vi "SOS main.vi"() -> ()   [LabVIEW 2017]
uses:
  <extravilib>/ChannelInstances/Lossy Stream-t'SSL Referee Game Status.ctl'.lvlib
  <extravilib>/ChannelInstances/Lossy Stream-t'AI Input.ctl'.lvlib
  SSL Referee Game Status.ctl
  SSL Detection Robot.ctl
  SSL Detection Ball.ctl
  SSL Detection Frame.ctl
  SSL/SSL Field State.ctl
  <extravilib>/ChannelInstances/Lossy Stream-t'SSL Field State.ctl'.lvlib
  <extravilib>/ChannelInstances/Lossy Stream-a[.](u8).lvlib
  <vilib>/Analysis/Matrix/Datatypes/RealMatrix.ctl
  <vilib>/Analysis/Matrix/NI_Matrix.lvlib
  <extravilib>/ChannelInstances/Lossy Stream-c(a[.](c(c(dbl,dbl,dbl,dbl,dbl),c(dbl,dbl,dbl,dbl,dbl),c(dbl,dbl,dbl,dbl,dbl,u32),u32,u32)),t'Events.ctl').lvlib
  <extravilib>/ChannelInstances/Lossy Stream-c(t'AI Ball.ctl',a[.](c(c(dbl,dbl,dbl,dbl,dbl),c(dbl,dbl,dbl,dbl,dbl),c(dbl,dbl,dbl,dbl,dbl,u32),u32,u32))).lvlib
  <extravilib>/ChannelInstances/Lossy Stream-a[.](i32).lvlib
  Filters/Estimadores.ctl
  Control/SSL UDP Address.ctl
  Control/File Player.ctl
  Control/SSL Data Control.ctl
  Intel/Command Enum.ctl
  DrawTargets.ctl
  grSim/grSim RobotReplacement.ctl
  grSim/grSim_BallReplacement.ctl
  Core/AI Ball.ctl
panel:
  in  "Tab Control 2":T1(tab)
  out "2D Picture":picture
  out "Kick Error Histogram":cluster{dbl[], dbl[]}(graph)
  out "Goalie Error Histogram":cluster{dbl[], dbl[]}(graph)
  out "Heatmap by ID":picture
  in  "ID":i32
  in  "Kalman Error\nID":i32
  out "Kalman Error Histogram":cluster{dbl[], dbl[]}(graph)
  in  "element":T3
  in  "grid y":dbl=30.0 format="%#_13g"
  in  "grid x":dbl=45.0 format="%#_13g"
  in  "Draw Targets?":T4={"Attacker"=TRUE, "Striker"=TRUE, "Goalie"=TRUE, "Defender"=TRUE, "kick"=TRUE, "Est Ball"=TRUE, "Est Robot"=FALSE}
  in  "SSL Data":T5={"Modo"=TRUE, "SSL UDP RX"={"Port:"=10020, "Server IP:"="224.5.23.2", "Local IP:"="", "RX"=TRUE}, "RefBox UDP RX"={"Port:"=10003, "Server IP:"="224.5.23.1", "Local IP:"="", "RX"=TRUE}, "Reprodução de Arquivo"={"file path (use dialog)"=path "E:/Media/2016-07-01_cmdragons_immortals.log", "size (in bytes)"=0, "offset (in bytes)"=0, "Slide"=0.0, "Play"=FALSE, "Time Stamp"=timestamp(0 s since 1904-01-01), "Playing"=FALSE}, "SSL UDP SOS RX IA_State"={"Port:"=10030, "Server IP:"="224.5.23.2", "Local IP:"="", "RX"=TRUE}, "SSL UDP SOS RX  Enemy State"={"Port:"=10020, "Server IP:"="224.5.23.2", "Local IP:"="224.5.23.2", "RX"=FALSE}} {"Reprodução de Arquivo"."Time Stamp" format="%<%.3X %x>T"; "Reprodução de Arquivo"."Slide" min=0 max=1 scale=0.0..1.0; "Reprodução de Arquivo"."offset (in bytes)" format="%.3p"; "Reprodução de Arquivo"."size (in bytes)" format="%.3p"}
  out "error out 5":errorcluster
  out "error out 3":errorcluster
  out "IA command":T8
  in  "ignora esquerda?":bool
  in  "ignora lado?":bool
  in  "Defense stretch":i32=300
  in  "Defense radius":i32=460
  in  "Estimador":T9=enum."Kalman"
  out "Total Delay":dbl format="%#.5g"
  in  "Goalie":string(combo)="0"
  in  "Command":string(combo)="Auto"
  in  "Time":enum16{"Azul", "Amarelo"}(ring) caption="Enum"
  in  "Lado":enum16{"Esquerdo", "Direito"}(ring) caption="Enum"
  in  "Tab Control":enum32{"RX Info", "TX info", "AI Parameters"}(tab)
  out "Game Status":T10={"Stage"="Normal First Half Pre", "Command"="Stop", "Time Left"=0.0, "Yellow Team"="", "Blue Team"="", "Yellow Score"=0, "Blue Score"=0, "Yellow Red Cards"=0, "Blue Red Cards"=0, "Yellow Yellow Cards"=0, "Blue Yellow Cards"=0, "Yellow Timeouts Left"=0, "Blue Timeouts Left"=0, "Yellow Timeout Remaining"=0.0, "Blue Timeout Remaining"=0.0, "Yellow Goalie Id"=0, "Blue Goalie Id"=0, "Time"=timestamp(2082758400 s since 1904-01-01)} {"Time" format="%<%.3X %x>T"; "Blue Timeout Remaining" format="%<%M:%S>t"; "Yellow Timeout Remaining" format="%<%M:%S>t"; "Time Left" format="%<%M:%S>t"}
  in  "Serial TX":bool
  in  "UDP TX":bool=TRUE
  in  "Address:":string="127.0.0.1"
  in  "Port:":u16=20011
  in  "Porta:":refnum<visa-resource-name>
  out "Comm FPS":dbl
  in  "replace active":bool
  in  "grSim replacement":cluster{"robots":T11[], "ball":T12}={"robots"=[{"x"=0.0, "y"=-450.0, "dir"=0.0, "yellowteam"=FALSE, "id"=0}, {"x"=0.0, "y"=-270.0, "dir"=0.0, "yellowteam"=FALSE, "id"=1}, {"x"=0.0, "y"=-90.0, "dir"=0.0, "yellowteam"=FALSE, "id"=2}, {"x"=0.0, "y"=90.0, "dir"=0.0, "yellowteam"=FALSE, "id"=3}, {"x"=0.0, "y"=270.0, "dir"=0.0, "yellowteam"=FALSE, "id"=4}, {"x"=0.0, "y"=450.0, "dir"=0.0, "yellowteam"=FALSE, "id"=5}], "ball"={"x"=0.0, "y"=0.0, "vx"=0.0, "vy"=0.0}}
  # "UDP"
  # "LOG"
  # "Score"
  # "Red Cards"
  # "Yellow Cards"
  # "Timeouts Left"
  # "Timeout Remaining"
  # "Goalie ID"
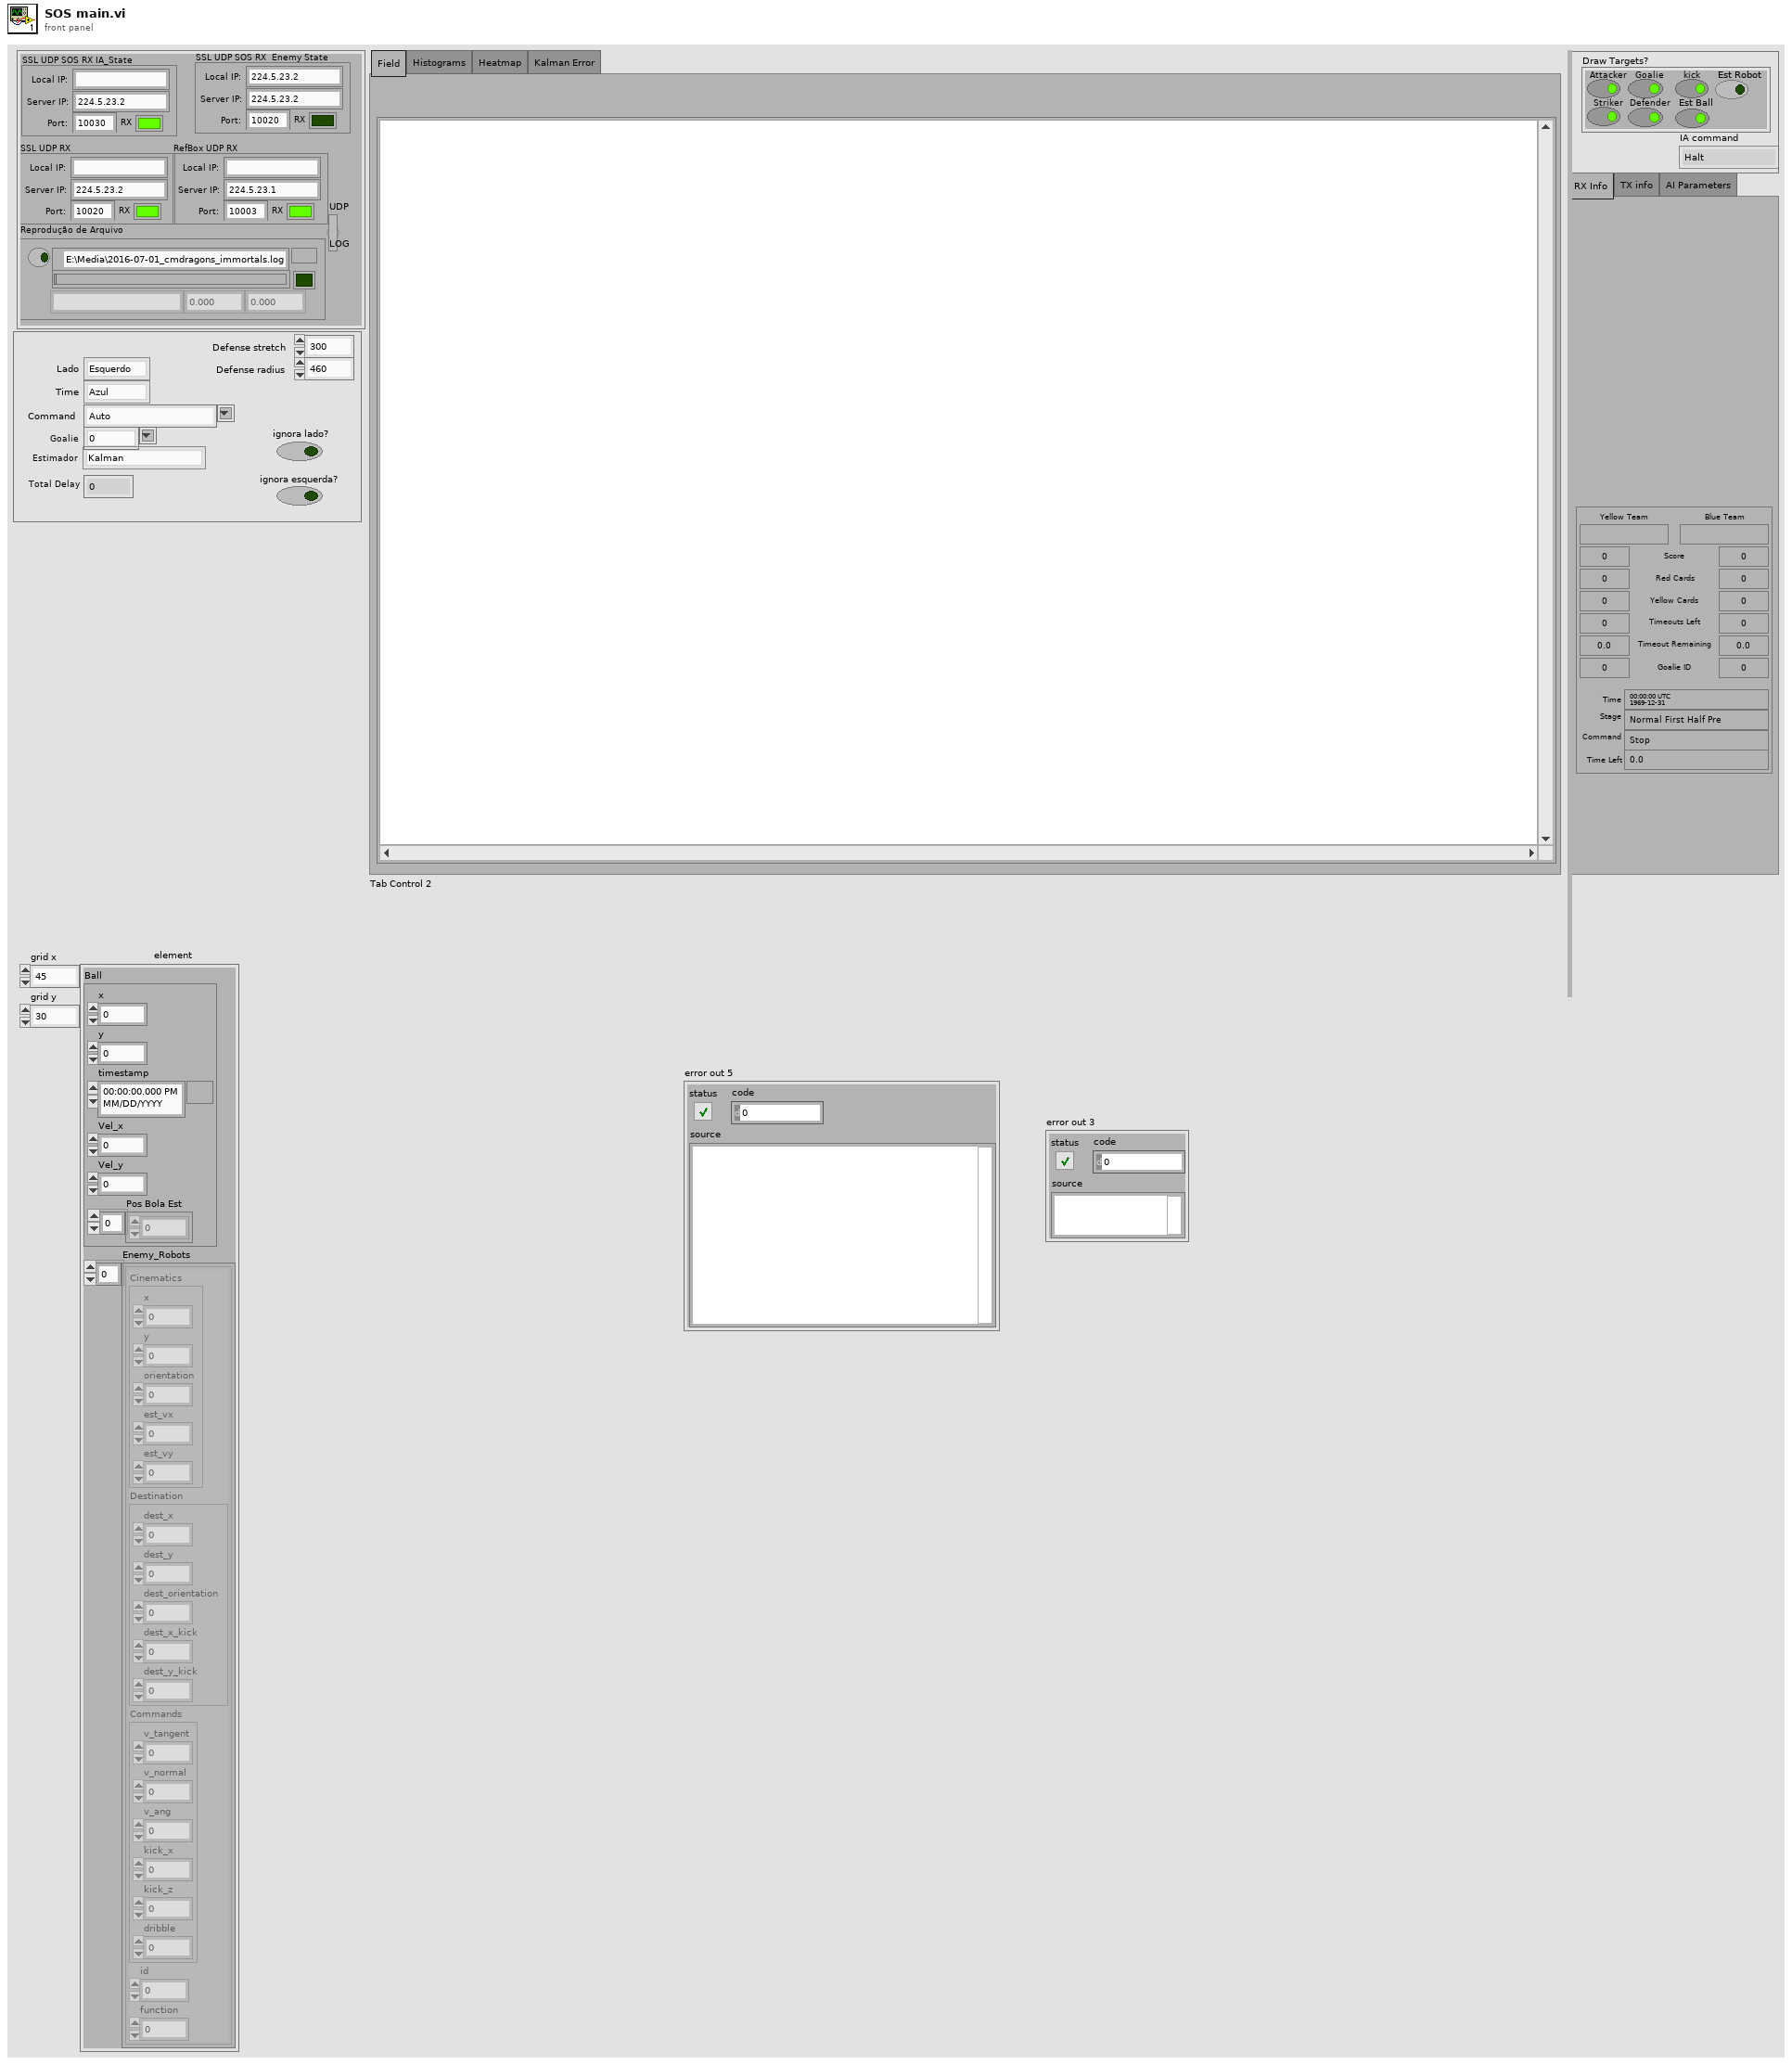
[diagram p1: front panel]
types:
  T1 = enum32{"Field", "Histograms", "Heatmap", "Kalman Error"}
  T2 = typedef "AI Ball.ctl" = cluster{"x":dbl, "y":dbl, "timestamp":timestamp, "Vel_x":dbl, "Vel_y":dbl, "Pos Bola Est":dbl[]}
  T3 = cluster{"Ball":T2, "Enemy_Robots":cluster{"Cinematics":cluster{"x":dbl, "y":dbl, "orientation":dbl, "est_vx":dbl, "est_vy":dbl}, "Destination":cluster{"dest_x":dbl, "dest_y":dbl, "dest_orientation":dbl, "dest_x_kick":dbl, "dest_y_kick":dbl}, "Commands":cluster{"v_tangent":dbl, "v_normal":dbl, "v_ang":dbl, "kick_x":dbl, "kick_z":dbl, "dribble":u32}, "id":u32, "function":u32}[]}
  T4 = typedef "DrawTargets.ctl" = cluster{"Attacker":bool, "Striker":bool, "Goalie":bool, "Defender":bool, "kick":bool, "Est Ball":bool, "Est Robot":bool}
  T5 = typedef "SSL Data Control.ctl" = cluster{"Modo":bool, "SSL UDP RX":T6, "RefBox UDP RX":T6, "Reprodução de Arquivo":T7, "SSL UDP SOS RX IA_State":T6, "SSL UDP SOS RX  Enemy State":T6}
  T6 = typedef "SSL UDP Address.ctl" = cluster{"Port:":u16, "Server IP:":string, "Local IP:":string, "RX":bool}
  T7 = typedef "File Player.ctl" = cluster{"file path (use dialog)":path, "size (in bytes)":i64, "offset (in bytes)":i64, "Slide":sgl, "Play":bool, "Time Stamp":timestamp, "Playing":bool}
  T8 = typedef "Command Enum.ctl" = enum16{"Halt", "Stop", "Force Start", "PKA Normal Start", "Prepare Kickoff Ally", "PKE Normal Start", "Prepare Kickoff Enemy", "Prepare Penalty Ally", "PPA Normal Start", "Prepare Penalty Enemy", "PPE Normal Start", "Direct Free Enemy", "Direct Free Ally", "Indirect Free Enemy", "Indirect Free Ally", "Timeout Enemy", "Timeout Ally", "Goal Enemy", "Goal Ally", "Ball Placement Enemy", "Ball Placement Ally", "Normal Half Time", "Extra Time Break", "Extra Half Time", "None", "Post Game"}
  T9 = typedef "Estimadores.ctl" = enum16{"Nenhum", "Simples", "Kalman"}
  T10 = typedef "SSL Referee Game Status.ctl" = cluster{"Stage":string, "Command":string, "Time Left":dbl, "Yellow Team":string, "Blue Team":string, "Yellow Score":u32, "Blue Score":u32, "Yellow Red Cards":u32, "Blue Red Cards":u32, "Yellow Yellow Cards":u32, "Blue Yellow Cards":u32, "Yellow Timeouts Left":u32, "Blue Timeouts Left":u32, "Yellow Timeout Remaining":dbl, "Blue Timeout Remaining":dbl, "Yellow Goalie Id":u32, "Blue Goalie Id":u32, "Time":timestamp}
  T11 = typedef "grSim RobotReplacement.ctl" = cluster{"x":dbl, "y":dbl, "dir":dbl, "yellowteam":bool, "id":u32}
  T12 = typedef "grSim_BallReplacement.ctl" = cluster{"x":dbl, "y":dbl, "vx":dbl, "vy":dbl}
  T13 = typedef "Lossy Stream-a[.](u8).lvlib/)Channel.ctl" = refnum<queue>
  T14 = typedef "Lossy Stream-c(t'AI Ball.ctl',a[.](c(c(dbl,dbl,dbl,dbl,dbl),c(dbl,dbl,dbl,dbl,dbl),c(dbl,dbl,dbl,dbl,dbl,u32),u32,u32))).lvlib/)Channel.ctl" = refnum<queue>
  T15 = typedef "SSL Field State.ctl" = cluster{"Detection Frame Out":T16, "Field Size Out":cluster{"line_width":u32, "field_length":u32, "field_width":u32, "boundary_width":u32, "referee_width":u32, "goal_width":u32, "goal_depth":u32, "goal_wall_width":u32, "center_circle_radius":u32, "defense_radius":u32, "defense_stretch":u32, "free_kick_from_defense_dist":u32, "penalty_spot_from_field_line_dist":u32, "penalty_line_from_spot_dist":u32}, "Received Time Stamp":timestamp}
  T16 = typedef "SSL Detection Frame.ctl" = cluster{"frame_number":u32, "t_capture":dbl, "t_sent":dbl, "camera_id":u32, "robots_yellow":T17[], "robots_blue":T17[], "balls":T19[], "Valid":bool, "Time Stamp":timestamp}
  T17 = typedef "SSL Detection Robot.ctl" = cluster{"x":sgl, "robot_id":u32, "confidence":sgl, "y":sgl, "orientation":sgl, "pixel_x":sgl, "pixel_y":sgl, "height":sgl, "Valid":bool, "Time Stamp":timestamp, "x_k|k":T18, "Pk|k":T18, "Previous Time Stamp":timestamp, "R":T18}
  T18 = typedef "NI_Matrix.lvlib/RealMatrix.ctl" = dbl[][]
  T19 = typedef "SSL Detection Ball.ctl" = cluster{"x":sgl, "area":u32, "confidence":sgl, "y":sgl, "z":sgl, "pixel_x":sgl, "pixel_y":sgl, "Valid":bool, "Time Stamp":timestamp, "x_k|k":T18, "Pk|k":T18, "Id":u32, "Previous Time Stamp":timestamp, "R":T18}
  T20 = cluster{"line_width":u32, "field_length":u32, "field_width":u32, "boundary_width":u32, "referee_width":u32, "goal_width":u32, "goal_depth":u32, "goal_wall_width":u32, "center_circle_radius":u32, "defense_radius":u32, "defense_stretch":u32, "free_kick_from_defense_dist":u32, "penalty_spot_from_field_line_dist":u32, "penalty_line_from_spot_dist":u32}
  T21 = typedef "Lossy Stream-t'SSL Field State.ctl'.lvlib/)Channel.ctl" = refnum<queue>
  T22 = typedef "Events.ctl" = cluster{"Touch":bool, "Ball out":bool, "id touch":dbl, "Ball out of \nVision":bool, "Ball inside \nGoalie area":bool, "Robot not responding":bool, "Robots responding status":dbl[], "Enemy Ball \nPossession":bool, "Pass State":bool, "id end of pass":dbl, "Kick":bool, "Id ini Possession":dbl, "Ball Possesion":bool, "Id Possesion":dbl}
  T23 = cluster{"Our_Robots":cluster{"Cinematics":cluster{"x":dbl, "y":dbl, "orientation":dbl, "est_vx":dbl, "est_vy":dbl}, "Destination":cluster{"dest_x":dbl, "dest_y":dbl, "dest_orientation":dbl, "dest_x_kick":dbl, "dest_y_kick":dbl}, "Commands":cluster{"v_tangent":dbl, "v_normal":dbl, "v_ang":dbl, "kick_x":dbl, "kick_z":dbl, "dribble":u32}, "id":u32, "function":u32}[], "Events":T22}
  T24 = typedef "Lossy Stream-c(a[.](c(c(dbl,dbl,dbl,dbl,dbl),c(dbl,dbl,dbl,dbl,dbl),c(dbl,dbl,dbl,dbl,dbl,u32),u32,u32)),t'Events.ctl').lvlib/)Channel.ctl" = refnum<queue>
  T25 = typedef "SSL Referee.ctl" = cluster{"packet_\ntimestamp":u64, "stage":u64, "stage_time_left":i32, "command ":u64, "command_\ncounter ":u32, "command_\ntimestamp":u64, "yellow team info":T26, "blue team info":T26, "Point":cluster{"x":sgl, "y":sgl}}
  T26 = typedef "SSL Referee Team Info.ctl" = cluster{"name":string, "score":u32, "red_cards":u32, "yellow_cards_time":u32[], "yellow_cards":u32, "timeout":u32, "timeout_times":u32, "goalie":u32}
  T27 = typedef "Lossy Stream-t'SSL Referee Game Status.ctl'.lvlib/)Channel.ctl" = refnum<queue>
  T28 = typedef "AI Input.ctl" = cluster{"our_robots":T29[], "enemy_robots":T29[], "balls":T2[], "geometry":T32, "IA Judge":T33, "Received Timestamp":timestamp, "Events":T22}
  T29 = typedef "AI Robot.ctl" = cluster{"id":u32, "function":T30, "x":dbl, "y":dbl, "orientation":dbl, "v_tangent":dbl, "v_normal":dbl, "v_ang":dbl, "kick_x":dbl, "kick_z":dbl, "dribble":bool, "Timestamp":timestamp, "dest_x":dbl, "dest_y":dbl, "dest_orientation":dbl, "estimatives":cluster{"est_v_tangent":dbl, "est_v_normal":dbl, "est_vx":dbl, "est_vy":dbl, "Pos Robot Est":dbl[]}, "dest_x_kick":dbl, "dest_y_kick":dbl, "Gap Coord":dbl[], "States":T31}
  T30 = typedef "Functions Enum.ctl" = enum16{"Attacker", "Goalie", "Defender", "Striker", "Goto 0", "Dummy", "Kicker", "ZigZag"}
  T31 = typedef "AttackerStates.ctl" = enum16{"Pass", "GoToTangent", "BallGetting", "GoToKick", ""}
  T32 = typedef "Field Size.ctl" = cluster{"line_width":u32, "field_length":u32, "field_width":u32, "boundary_width":u32, "referee_width":u32, "goal_width":u32, "goal_depth":u32, "goal_wall_width":u32, "center_circle_radius":u32, "defense_radius":u32, "defense_stretch":u32, "free_kick_from_defense_dist":u32, "penalty_spot_from_field_line_dist":u32, "penalty_line_from_spot_dist":u32}
  T33 = typedef "AI Judge.ctl" = cluster{"stage":string, "command":string, "our_goalie_id":dbl, "enemy_goalie_id":dbl, "command enum":T8, "Time":enum16{"Azul", "Amarelo"}}
  T34 = typedef "Lossy Stream-a[.](i32).lvlib/)Channel.ctl" = refnum<queue>
  T35 = typedef "Lossy Stream-t'AI Input.ctl'.lvlib/)Channel.ctl" = refnum<queue>
  T36 = typedef "grSim Robot Command.ctl" = cluster{"id":u32, "kickspeedx":sgl, "kickspeedz":sgl, "veltangent":sgl, "velnormal":sgl, "velangular":sgl, "spinner":bool, "wheelspeed":bool, "wheel1":sgl, "wheel2":sgl, "wheel3":sgl, "wheel4":sgl}
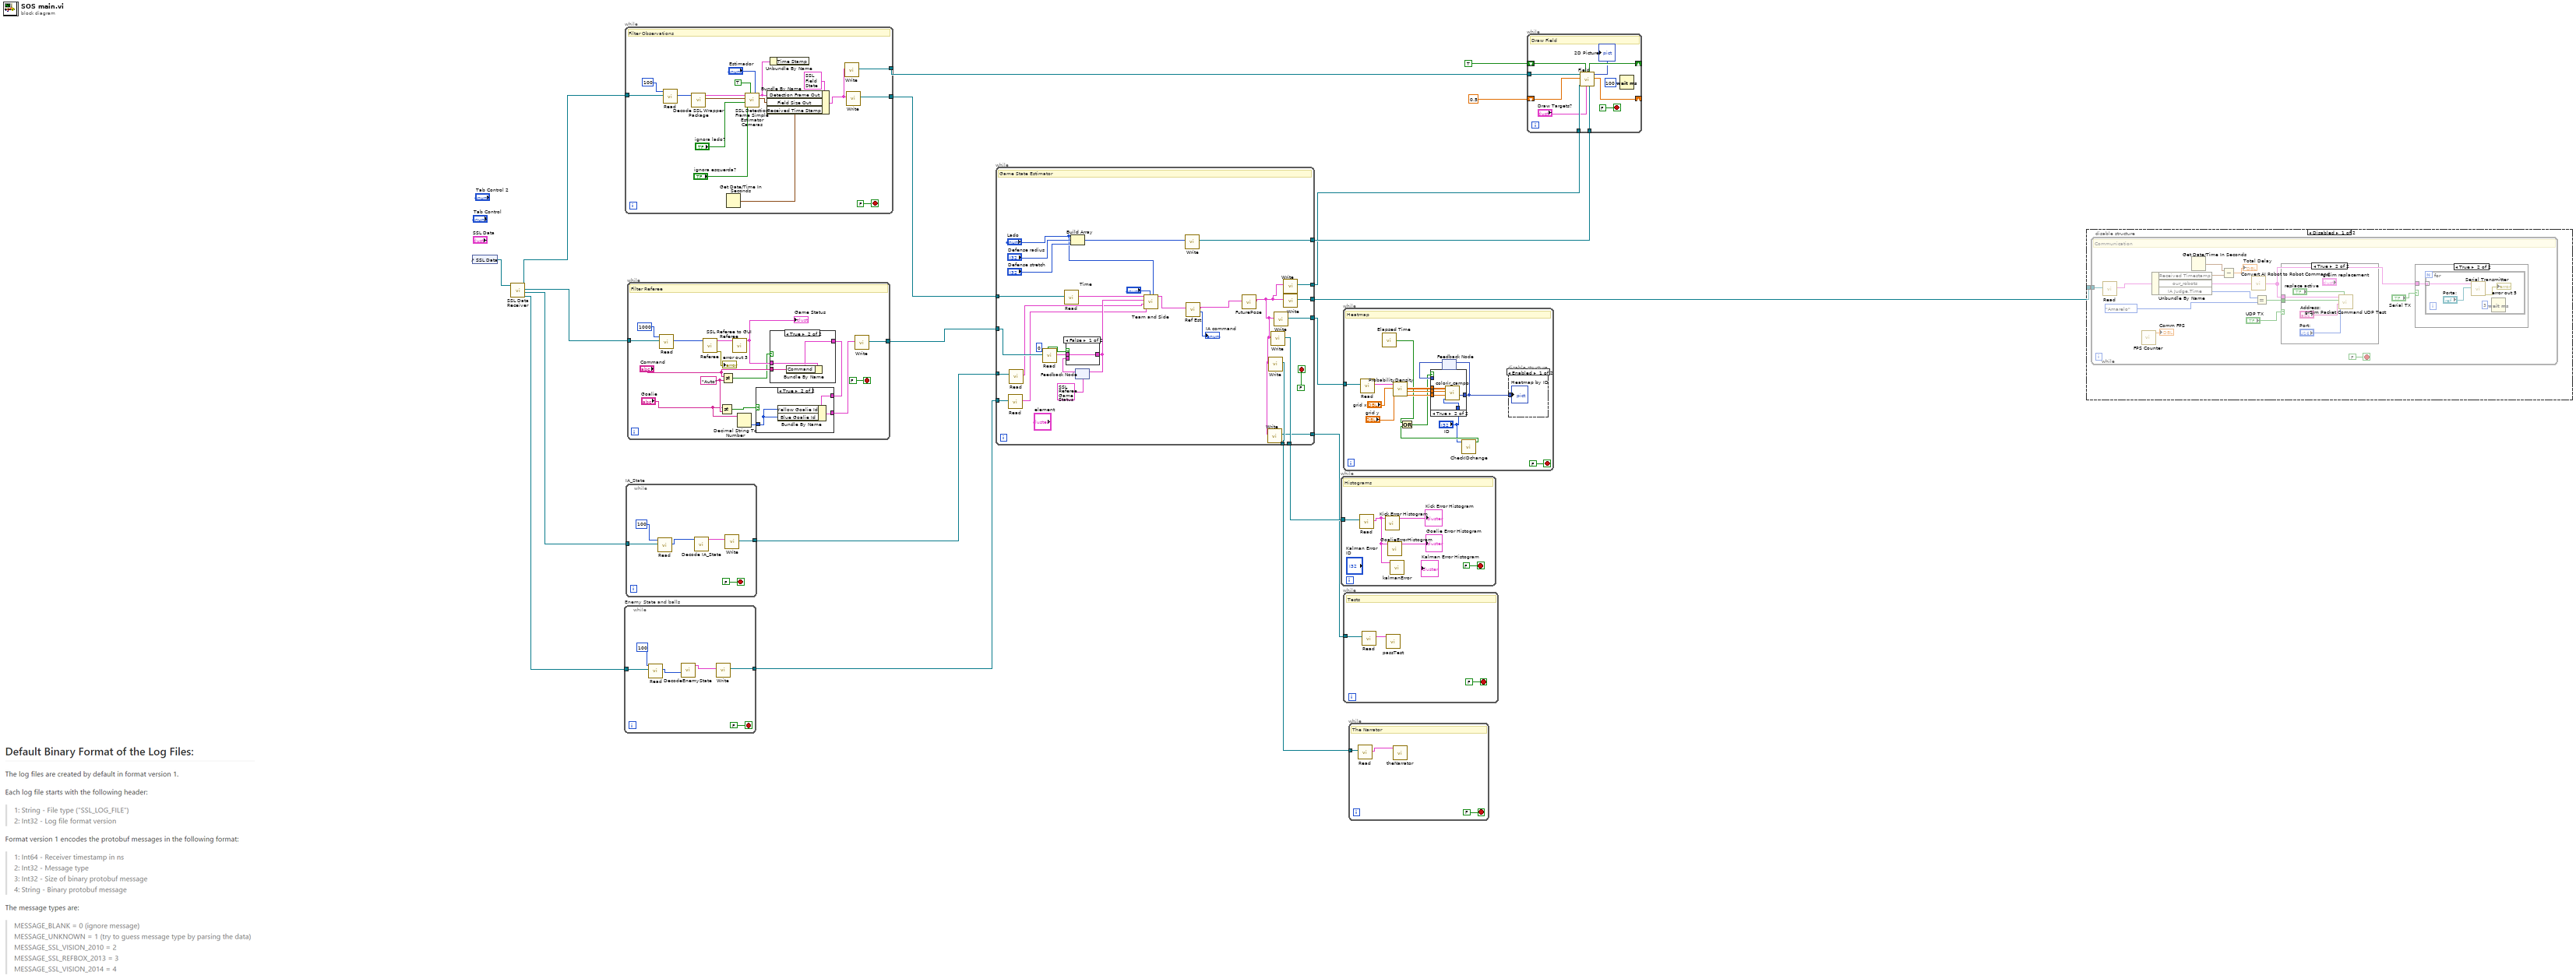
[diagram p0: block diagram]
diagram:
  n1 = control-ref of="SSL Data"() -> (w9:refnum<vi>)
  n2 = call "SSL Data Receiver.vi"("SSL Data"=w9) -> ("Enemy_State"=w10:T13, "IA_State"=w11:T13, "SSL RefBox"=w14:T13, "SSL Vision"=w15:T13)  [unwired: 7 in]
  n3 = while "Enemy State and balls" {
    tunnel: w10 -> [w23]
    tunnel: [w20] -> w7
    stop <- FALSE stop-if-true
    n4 = call <extravilib>:"Read.vi"("channel"=w23, "timeout in ms (-1)"=100) -> ("element"=w24:u8[])  [unwired: 4 in, 5 out]
    n5 = call "DecodeEnemyState.vi"("array"=w24) -> ("output cluster"=w21:T3)  [unwired: 8 in, 2 out]
    n6 = call <extravilib>:"Write.vi"("element"=w21) -> ("channel"=w20:T14)  [unwired: 8 in, 2 out]
  }
  n7 = while {
    tunnel: [w27] -> w13
    tunnel: [w35] -> w17
    tunnel: w15 -> [w32]
    stop <- FALSE stop-if-true
    # "Filter Observations"
    n8 = call <extravilib>:"Read.vi"("channel"=w32, "timeout in ms (-1)"=100) -> ("element"=w31:u8[])  [unwired: 4 in, 5 out]
    n9 = call "Decode SSL Wrapper Package.vi"("unsigned byte array"=w31) -> ("Field Size"=w40:T20, "Detection Frame"=w41:T16)  [unwired: 7 in, 2 out]
    n10 = Get Date/Time In Seconds() -> (seconds since 1Jan1904=w37:timestamp)
    n11 = call "SSL Detection Frame Simple Estimator Cameras.vi"("Estimador"="Estimador", "Enable"=TRUE, "ignora esquerda?"="ignora esquerda?", "ignora lado?"="ignora lado?", "Field Size"=w40, "Detection Frame In"=w41) -> ("Field Size Out"=w36:T20, "Detection Frame Out"=w34:T16)  [unwired: 4 in]
    n12 = Bundle By Name(cluster=T15 {"Detection Frame Out"={"frame_number"=0, "t_capture"=0.0, "t_sent"=0.0, "camera_id"=0, "robots_yellow"=[], "robots_blue"=[], "balls"=[], "Valid"=FALSE, "Time Stamp"=timestamp(0 s since 1904-01-01)}, "Field Size Out"={"line_width"=0, "field_length"=0, "field_width"=0, "boundary_width"=0, "referee_width"=0, "goal_width"=0, "goal_depth"=0, "goal_wall_width"=0, "center_circle_radius"=0, "defense_radius"=0, "defense_stretch"=0, "free_kick_from_defense_dist"=0, "penalty_spot_from_field_line_dist"=0, "penalty_line_from_spot_dist"=0}, "Received Time Stamp"=timestamp(0 s since 1904-01-01)}, "Detection Frame Out"=w34, "Field Size Out"=w36, "Received Time Stamp"=w37) -> (w26:T15)
    n13 = Unbundle By Name(w34) -> ()  [unwired: 1 out]
    n14 = call <extravilib>:"Write.vi"("element"=w26) -> ("channel"=w27:T21)  [unwired: 8 in, 2 out]
    n15 = call <extravilib>:"Write.vi"("element"=w26) -> ("channel"=w35:T21)  [unwired: 8 in, 2 out]
  }
  n16 = while "IA_State" {
    tunnel: w11 -> [w47]
    tunnel: [w43] -> w8
    stop <- FALSE stop-if-true
    n17 = call <extravilib>:"Read.vi"("channel"=w47, "timeout in ms (-1)"=100) -> ("element"=w45:u8[])  [unwired: 4 in, 5 out]
    n18 = call "Decode IA_State.vi"("array"=w45) -> ("output cluster"=w44:T23)  [unwired: 9 in, 1 out]
    n19 = call <extravilib>:"Write.vi"("element"=w44) -> ("channel"=w43:T24)  [unwired: 8 in, 2 out]
  }
  n20 = while {
    tunnel: w14 -> [w51]
    tunnel: [w61] -> w16
    stop <- FALSE stop-if-true
    w57 = "Auto" ("y")
    # "Filter Referee"
    n21 = call <extravilib>:"Read.vi"("channel"=w51, "timeout in ms (-1)"=1000) -> ("element"=w50:u8[])  [unwired: 4 in, 5 out]
    n22 = call "Referee.vi"("element"=w50) -> ("output cluster"=w62:T25, "error out"=→"error out 3":errorcluster)  [unwired: 13 in]
    n23 = Not Equal?(x="Goalie", y=w57) -> (x != y?=w56:bool)
    n24 = Not Equal?(x="Command", y=w57) -> (x != y?=w58:bool)
    n25 = call "SSL Referee to GUI Referee.vi"("SSL Game Status"=w62) -> ("GUI Game Status"=w60:T10)  [unwired: 10 in]
    "Game Status" <- w60
    n26 = Decimal String To Number(string="Goalie") -> (number=w52:i32)  [unwired: 2 in, 1 out]
    n27 = case shown="True" w58 {
      tunnel: w60 -> [w69 w72]
      tunnel: [w69 w71] -> w55
      tunnel: "Command" -> [_ w70]
      frame False {
      }
      frame True {
        n28 = Bundle By Name(cluster=w72, "Command"=w70) -> (w71:T10)
      }
    }
    n29 = case shown="True" w56 {
      tunnel: w55 -> [w65 w68]
      tunnel: [w65 w67] -> w54
      tunnel: w52 -> [_ w66]
      frame False {
      }
      frame True {
        n30 = Bundle By Name(cluster=w68, "Yellow Goalie Id"=w66, "Blue Goalie Id"=w66) -> (w67:T10)
      }
    }
    n31 = call <extravilib>:"Write.vi"("element"=w54) -> ("channel"=w61:T27)  [unwired: 8 in, 2 out]
  }
  n32 = while {
    tunnel: w17 -> [w78]
    tunnel: w16 -> [w101]
    tunnel: [w95] -> w6
    tunnel: [w80] -> w12
    tunnel: [w88] -> w5
    tunnel: w8 -> [w87]
    tunnel: w7 -> [w86]
    tunnel: [w81] -> w4
    tunnel: [w76] -> w3
    tunnel: [w75] -> w2
    tunnel: [w73] -> w1
    stop <- FALSE stop-if-true
    # "Game State Estimator"
    n33 = call <extravilib>:"Read.vi"("channel"=w86) -> ("element"=w84:T3)  [unwired: 5 in, 5 out]
    n34 = call <extravilib>:"Read.vi"("channel"=w87) -> ("element"=w85:T23)  [unwired: 5 in, 5 out]
    n35 = call <extravilib>:"Read.vi"("channel"=w101, "timeout in ms (-1)"=0) -> ("element"=w98:T10, "timed out?"=w99:bool)  [unwired: 4 in, 4 out]
    n36 = call <extravilib>:"Read.vi"("channel"=w78) -> ("element"=w77:T15)  [unwired: 5 in, 5 out]
    n37 = Build Array("Lado", "Defense radius", "Defense stretch") -> (w79:i32[])
    n38 = feedback #1(T10 {"Stage"="First Half", "Command"="Stop", "Time Left"=0.0, "Yellow Team"="", "Blue Team"="", "Yellow Score"=0, "Blue Score"=0, "Yellow Red Cards"=0, "Blue Red Cards"=0, "Yellow Yellow Cards"=0, "Blue Yellow Cards"=0, "Yellow Timeouts Left"=0, "Blue Timeouts Left"=0, "Yellow Timeout Remaining"=0.0, "Blue Timeout Remaining"=0.0, "Yellow Goalie Id"=0, "Blue Goalie Id"=0, "Time"=timestamp(0 s since 1904-01-01)} ("element")) -> (w97:T10)
    n39 = case shown="False" w99 {
      tunnel: w98 -> [w103 _]
      tunnel: [w103 w104] -> w96
      tunnel: w97 -> [_ w104]
      frame False {
      }
      frame True {
      }
    }
    n40 = feedback-in #1(w96) -> ()
    n41 = call "Team and Side.vi"("Lado"="Lado", "Time"="Time", "Enemy state and balls"=w84, "IA_State"=w85, "Game Status"=w96, "Field State Input"=w77) -> ("IA State"=w83:T28)  [unwired: 5 in]
    n42 = call <extravilib>:"Write.vi"("element"=w79) -> ("channel"=w80:T34)  [unwired: 8 in, 2 out]
    n43 = call "Ref Est.vi"("IA State Input"=w83) -> ("IA command"=→"IA command":T8, "IA State Output"=w82:T28)  [unwired: 9 in]
    n44 = call "FuturePose.vi"("IA State Input"=w82) -> ("output cluster"=w74:T28)  [unwired: 10 in]
    n45 = call <extravilib>:"Write.vi"("element"=w74) -> ("channel"=w73:T35)  [unwired: 8 in, 2 out]
    n46 = call <extravilib>:"Write.vi"("element"=w74) -> ("channel"=w75:T35)  [unwired: 8 in, 2 out]
    n47 = call <extravilib>:"Write.vi"("element"=w74) -> ("channel"=w76:T35)  [unwired: 8 in, 2 out]
    n48 = call <extravilib>:"Write.vi"("element"=w74) -> ("channel"=w81:T35)  [unwired: 8 in, 2 out]
    n49 = call <extravilib>:"Write.vi"("element"=w74) -> ("channel"=w88:T35)  [unwired: 8 in, 2 out]
    n50 = call <extravilib>:"Write.vi"("element"=w74) -> ("channel"=w95:T35)  [unwired: 8 in, 2 out]
  }
  n51 = while {
    tunnel: w3 -> [w108]
    stop <- FALSE stop-if-true
    # "Histograms"
    n52 = call <extravilib>:"Read.vi"("channel"=w108) -> ("element"=w105:T28)  [unwired: 5 in, 5 out]
    n53 = call "Kick Error Histogram.vi"("IA state"=w105) -> ("Kick Error Histogram"=→"Kick Error Histogram":cluster{dbl[], dbl[]})  [unwired: 10 in]
    n54 = call "GoalieErrorHistogram.vi"("IA state"=w105) -> ("Goalie Error Histogram"=→"Goalie Error Histogram":cluster{dbl[], dbl[]})  [unwired: 10 in]
    n55 = call "kalmanError.vi"("IA state"=w105) -> ()  [unwired: 11 in]
  }
  n56 = while {
    tunnel: w4 -> [w116]
    stop <- FALSE stop-if-true
    # "Heatmap"
    n57 = call <extravilib>:"Read.vi"("channel"=w116) -> ("element"=w117:T28)  [unwired: 5 in, 5 out]
    n58 = call "Elapsed Time"() -> ("Time has Elapsed"=w112:bool)  [unwired: 12 in, 7 out]
    n59 = call "ProbabilityDensity.vi"("grid y"="grid y", "grid x"="grid x", "IA state"=w117) -> ("grid y out"=w118:dbl, "grid x out"=w119:dbl, "3D Probability Matrix"=w120:dbl[][][])  [unwired: 6 in]
    n60 = feedback #2() -> (w114:picture)  [unwired: 1 in]
    n61 = call "CheckIDchange.vi"("ID"="ID") -> ("ID change"=w113:bool)  [unwired: 10 in]
    n62 = Or(x=w112, y=w113) -> (x .or. y?=w111:bool)
    n63 = case shown="True" w111 {
      tunnel: w120 -> [_ w129]
      tunnel: w119 -> [_ w128]
      tunnel: w118 -> [_ w127]
      tunnel: [w124 w126] -> w115
      tunnel: "ID" -> [_ w125]
      tunnel: w114 -> [w124 _]
      frame False {
      }
      frame True {
        n64 = call "colorir_campo.vi"("ID"=w125, "grid y"=w127, "grid x"=w128, "3D Probability Matrix"=w129) -> ("campo colorido"=w126:picture)  [unwired: 7 in]
      }
    }
    n65 = feedback-in #2(w115) -> ()
    n66 = disable-structure shown="Enabled" {
      disable-tunnel: w115 -> [w130 _]
      frame Enabled {
        "Heatmap by ID" <- w130
      }
      frame Disabled {
      }
    }
  }
  n67 = while {
    tunnel: w1 -> [w132]
    stop <- FALSE stop-if-true
    # "Tests"
    n68 = call <extravilib>:"Read.vi"("channel"=w132) -> ("element"=w131:T28)  [unwired: 5 in, 5 out]
    n69 = call "passTest.vi"("IA state"=w131) -> ()  [unwired: 11 in]
  }
  n70 = while {
    tunnel: w2 -> [w135]
    stop <- FALSE stop-if-true
    # "The Narrator"
    n71 = call <extravilib>:"Read.vi"("channel"=w135) -> ("element"=w134:T28)  [unwired: 5 in, 5 out]
    n72 = call "theNarrator.vi"("IA state"=w134) -> ()  [unwired: 11 in]
  }
  n73 = while {
    shift-right: [w146] -> _
    shift-left: 0.5 ("New Scale") -> [w141]
    shift-right: [w145] -> _
    shift-left: TRUE ("AutoScale Out") -> [w144]
    tunnel: w5 -> [w142]
    tunnel: w13 -> [w138]
    tunnel: w12 -> [w140]
    stop <- FALSE stop-if-true
    # "Draw Field"
    n74 = call "Field.vi"("channel 2"=w140, "Draw Targets?"="Draw Targets?", "AutoScale"=w144, "channel for IA State"=w142, "Scale mm/pixel"=w141, "channel"=w138) -> ("Scale Out"=w146:dbl, "2D Picture"=→"2D Picture":picture, "AutoScale Out"=w145:bool)  [unwired: 3 in]
    n75 = Wait (ms)(milliseconds to wait=u32 100) -> ()  [unwired: 1 out]
  }
  n76 = disable-structure shown="Disabled" {
    disable-tunnel: w6 -> [w148 _]
    frame Disabled {
      n77 = while {
        tunnel: w148 -> [w161]
        stop <- FALSE stop-if-true
        # "Communication"
        n78 = call <extravilib>:"Read.vi"("channel"=w161) -> ("element"=w160:T28)  [unwired: 5 in, 5 out]
        n79 = call "FPS Counter.vi"() -> ("Numeric"=→"Comm FPS":dbl)  [unwired: 11 in]
        n80 = Unbundle By Name(w160) -> ("Received Timestamp"=w155:timestamp, "our_robots"=w159:T29[], "IA Judge.Time"=w158:enum16{"Azul", "Amarelo"})
        n81 = Get Date/Time In Seconds() -> (seconds since 1Jan1904=w154:timestamp)
        n82 = Subtract(x=w154, y=w155) -> (x-y=→"Total Delay":dbl)
        n83 = call "Convert AI Robot to Robot Command.vi"("Input Array"=w159) -> ("Output Array"=w152:T36[])
        n84 = Equal?(x=w158, y=enum16{"Azul", "Amarelo"}."Amarelo") -> (x = y?=w156:bool)
        n85 = case shown="True" "UDP TX" {
          tunnel: w156 -> [_ w172]
          tunnel: w152 -> [_ w170]
          frame False {
          }
          frame True {
            n86 = call "grSim Packet Command UDP Test.vi"("replace ball"="replace active", "Port:"="Port:", "SSL Vision Address:"="Address:", "isteamyellow"=w172, "Robots"=w170) -> ()  [unwired: 7 in]
          }
        }
        n87 = case shown="True" "Serial TX" {
          tunnel: w152 -> [_ w163]
          frame False {
          }
          frame True {
            n88 = for {
              tunnel: w163 -> [w167] mode=indexing
              n89 = call "Serial Transmitter.vi"("Porta:"="Porta:", "Robots"=w167) -> ("error out"=→"error out 5":errorcluster)  [unwired: 9 in]
              n90 = Wait (ms)(milliseconds to wait=u32 3) -> ()  [unwired: 1 out]
            }
          }
        }
      }
    }
    frame Enabled {
    }
  }
